vi "EDS test 01_with motor and Firebase.vi"() -> ()   [LabVIEW 2020]
uses:
  <vilib>/Instr/_visa.llb/VISA Configure Serial Port (Instr).vi
  <vilib>/httpClient/PUTBuffer.vi
  <vilib>/httpClient/LabVIEWHTTPClient.lvlib
panel:
  out "Train Speed":string
  out "Trolley Speed":string
  out "Trolley Distance":dbl
  out "Elephant Distance":dbl
  out "error out":errorcluster
  in  "IR Sensor":bool
  out "concatenated string":string
  out "read buffer":string
  in  "stop":bool
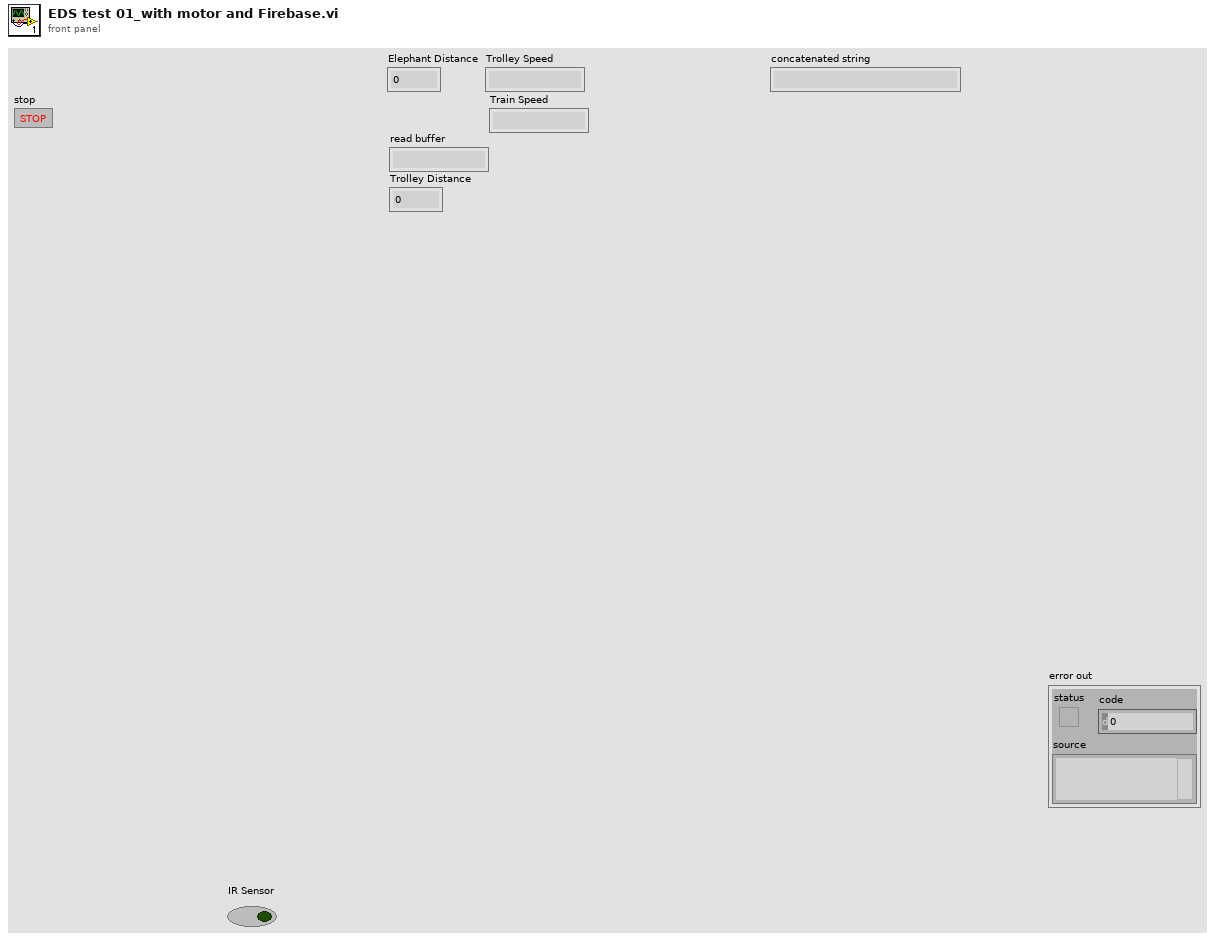
[diagram p1: front panel]
types:
  T1 = typedef "LabVIEWHTTPClient.lvlib/ClientHandle.ctl" = refnum<k1>
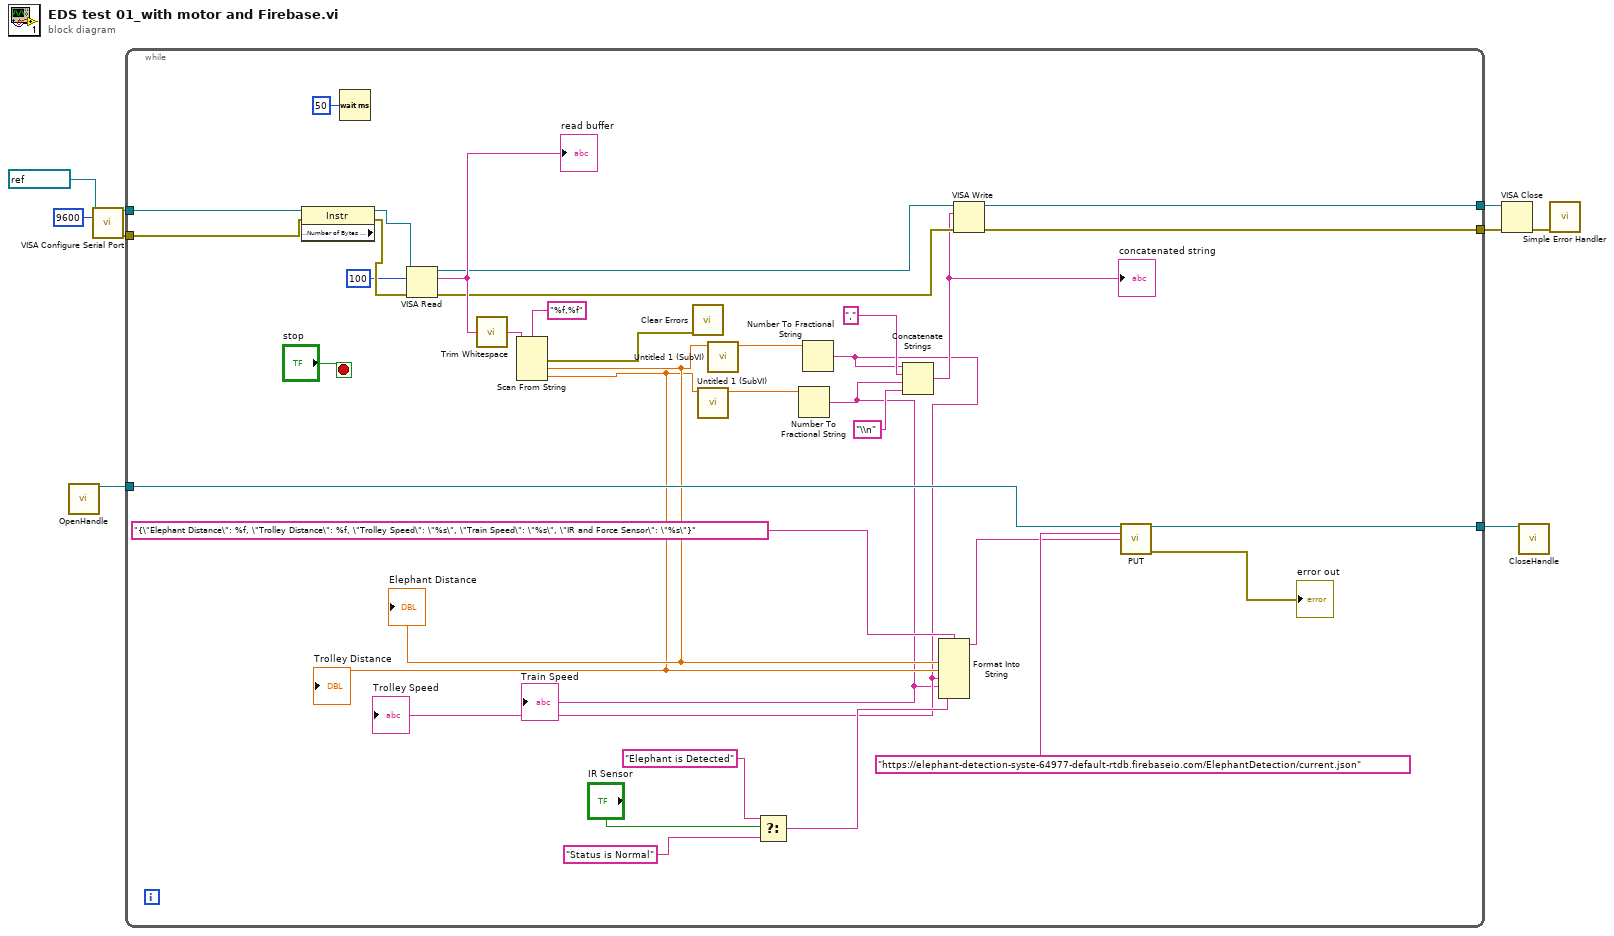
[diagram p0: block diagram]
diagram:
  n1 = call <vilib>:"OpenHandle.vi"() -> ("client handle out"=w2:T1)  [unwired: 14 in, 1 out]
  n2 = call-poly "VISA Configure Serial Port"("VISA resource name"=refnum<visa-resource-name> "COM3", "baud rate (9600)"=u32 9600) -> ("VISA resource name out"=w7:refnum<visa-resource-name>, "error out"=w6:errorcluster)  [unwired: 12 in]
  n3 = while {
    tunnel: w7 -> [w43]
    tunnel: w6 -> [w42]
    tunnel: [w28] -> w4
    tunnel: [w27] -> w3
    tunnel: w2 -> [w15]
    tunnel: [w14] -> w1
    stop <- "stop" stop-if-true
    n4 = property class="Instr" props=["Serial Settings:Number of Bytes at Serial Port"](reference=w43, error in=w42) -> (reference out=w38:refnum<visa-resource-name>, error out=w39:errorcluster)  [unwired: 1 out]
    n5 = Wait (ms)(milliseconds to wait=u32 50) -> ()  [unwired: 1 out]
    n6 = VISA Read(VISA resource name=w38, byte count=u32 100, error in (no error)=w39) -> (VISA resource name out=w30:refnum<visa-resource-name>, read buffer=w37:string, error out=w29:errorcluster)  [unwired: 1 out]
    "read buffer" <- w37
    n7 = call <vilib>:"Trim Whitespace.vi"("string"=w37) -> ("trimmed string"=w36:string)  [unwired: 1 in]
    n8 = Scan From String(format string="%f,%f", input string=w36) -> (error out=w34:errorcluster, output 1=w13:dbl, output 2=w12:dbl)  [unwired: 4 in, 2 out]
    "Elephant Distance" <- w13
    "Trolley Distance" <- w12
    n9 = call <vilib>:"Clear Errors.vi"("error in (no error)"=w34) -> ()  [unwired: 5 in, 2 out]
    n10 = call "Untitled 1 (SubVI).vi"("Ultrasonic 01"=w12) -> ("Numeric"=w31:dbl)  [unwired: 10 in]
    n11 = call "Untitled 1 (SubVI).vi"("Ultrasonic 01"=w13) -> ("Numeric"=w32:dbl)  [unwired: 10 in]
    n12 = Select(t="Elephant is Detected" ("format string"), s="IR Sensor", f="Status is Normal" ("format string")) -> (s? t:f=w20:string)
    n13 = Number To Fractional String(number=w31) -> (F-format string=w10:string)  [unwired: 3 in]
    "Train Speed" <- w10
    n14 = Number To Fractional String(number=w32) -> (F-format string=w11:string)  [unwired: 3 in]
    "Trolley Speed" <- w11
    n15 = Concatenate Strings(w11, ",", w10, "\\n") -> (w26:string)
    "concatenated string" <- w26
    n16 = Format Into String(format string="{\"Elephant Distance\": %f, \"Trolley Distance\": %f, \"Trolley Speed\": \"%s\", \"Train Speed\": \"%s\", \"IR and Force Sensor\": \"%s\"}", w13, w12, w11, w10, w20) -> (resulting string=w17:string)  [unwired: 2 in, 1 out]
    n17 = VISA Write(VISA resource name=w30, write buffer=w26, error in (no error)=w29) -> (VISA resource name out=w28:refnum<visa-resource-name>, error out=w27:errorcluster)  [unwired: 1 out]
    n18 = call-poly <vilib>:"PUT.vi"("client handle"=w15, "url"="https://elephant-detection-syste-64977-default-rtdb.firebaseio.com/ElephantDetection/current.json", "buffer"=w17) -> ("client handle out"=w14:T1, "error out"=→"error out":errorcluster)  [unwired: 9 in, 2 out]
  }
  n19 = VISA Close(VISA resource name=w4, error in (no error)=w3) -> (error out=w5:errorcluster)
  n20 = call <vilib>:"CloseHandle.vi"("client handle"=w1) -> ()  [unwired: 14 in, 1 out]
  n21 = call <vilib>:"Simple Error Handler.vi"("error in (no error)"=w5) -> ()  [unwired: 4 in, 5 out]
